vi "pseudoPath_gLocalizedPseudoPaths.vi"() -> ()   [LabVIEW 2016]
panel:
  in  "Localized osdatadir":string="<osdatadir>" caption="本地化系统数据目录"
  in  "DNL_nonlocalized pseudo paths":string[](array[string])=["<topvi>", "<foundvi>", "<vilib>", "<userlib>", "<instrlib>", "<osdatadir>"]
  in  "Localized pseudo paths":string[](array[string])=["<topvi>", "<foundvi>", "<vilib>", "<userlib>", "<instrlib>", "<osdatadir>"] caption="本地伪路径"
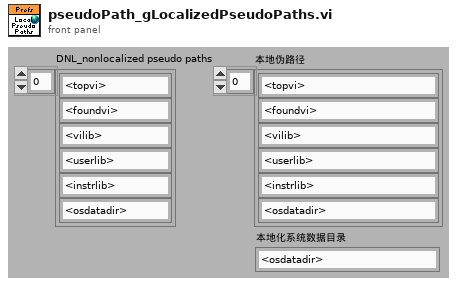
[diagram p1: front panel]
diagram:
